vi "Tanques.vi"() -> ()   [LabVIEW 2017]
panel:
  out "Alarma 3":bool
  out "Alarma 2":bool
  out "Alarma 1":bool
  out "Tank 1":i64(slide) scale=0.0..100.0
  out "Tank 3":i64(slide) scale=0.0..100.0
  out "Tank 2":i64(slide) scale=0.0..100.0
  out "Tank":i64(slide) scale=0.0..300.0
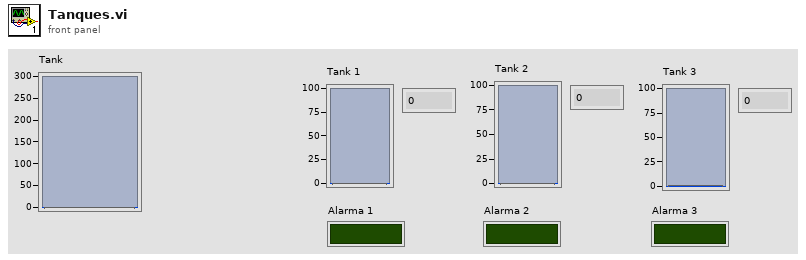
[diagram p1: front panel]
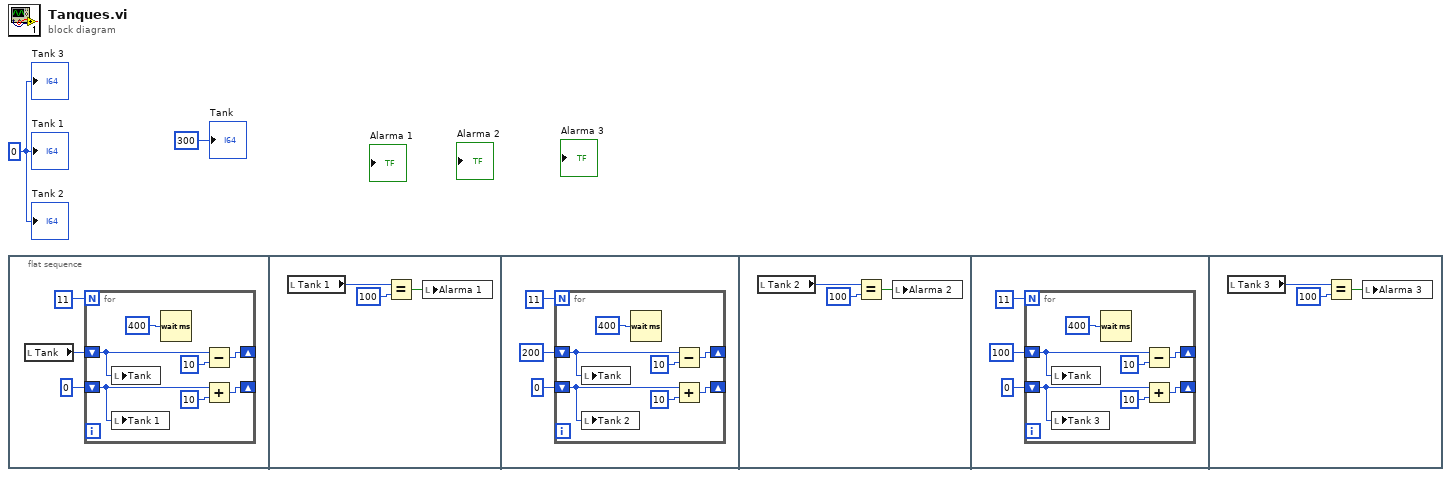
[diagram p0: block diagram]
diagram:
  w1 = i64 0 ("Tank 2")
  n1 = flat-sequence {
    frame #0 {
      n2 = local read "Tank"() -> (w3:i64)
      n3 = for {
        N: 11 -> [_]
        shift-right: [w11] -> _
        shift-left: i64 0 -> [w7]
        shift-right: [w9] -> _
        shift-left: w3 -> [w8]
        n4 = local write "Tank"(w8) -> ()
        n5 = local write "Tank 1"(w7) -> ()
        n6 = Wait (ms)(milliseconds to wait=u32 400) -> ()  [unwired: 1 out]
        n7 = Subtract(x=w8, y=i64 10) -> (x-y=w9:i64)
        n8 = Add(x=w7, y=i64 10) -> (x+y=w11:i64)
      }
    }
    frame #1 {
      n9 = local read "Tank 1"() -> (w13:i64)
      n10 = Equal?(x=w13, y=i64 100) -> (x = y?=w14:bool)
      n11 = local write "Alarma 1"(w14) -> ()
    }
    frame #2 {
      n12 = for {
        N: 11 -> [_]
        shift-right: [w23] -> _
        shift-left: i64 0 -> [w24]
        shift-right: [w21] -> _
        shift-left: i64 200 -> [w20]
        n13 = local write "Tank"(w20) -> ()
        n14 = local write "Tank 2"(w24) -> ()
        n15 = Wait (ms)(milliseconds to wait=u32 400) -> ()  [unwired: 1 out]
        n16 = Subtract(x=w20, y=i64 10) -> (x-y=w21:i64)
        n17 = Add(x=w24, y=i64 10) -> (x+y=w23:i64)
      }
    }
    frame #3 {
      n18 = local read "Tank 2"() -> (w26:i64)
      n19 = Equal?(x=w26, y=i64 100) -> (x = y?=w28:bool)
      n20 = local write "Alarma 2"(w28) -> ()
    }
    frame #4 {
      n21 = for {
        N: 11 -> [_]
        shift-right: [w37] -> _
        shift-left: i64 0 -> [w34]
        shift-right: [w32] -> _
        shift-left: i64 100 -> [w33]
        n22 = local write "Tank"(w33) -> ()
        n23 = local write "Tank 3"(w34) -> ()
        n24 = Wait (ms)(milliseconds to wait=u32 400) -> ()  [unwired: 1 out]
        n25 = Subtract(x=w33, y=i64 10) -> (x-y=w32:i64)
        n26 = Add(x=w34, y=i64 10) -> (x+y=w37:i64)
      }
    }
    frame #5 {
      n27 = local read "Tank 3"() -> (w41:i64)
      n28 = Equal?(x=w41, y=i64 100) -> (x = y?=w39:bool)
      n29 = local write "Alarma 3"(w39) -> ()
    }
  }
  "Tank" <- i64 300 ("Tank")
  "Tank 2" <- w1
  "Tank 3" <- w1
  "Tank 1" <- w1
